vi "Instantiate_llm_azureopenai.vi"(0 "deployement name":string(combo), 5 "azure_endpoint":string, 7 "azure_api_key":string, 9 "api_version":string, 11 "error in (no error)":errorcluster) -> (4 "llm_azureopenai_chatmodels out":refnum<class "llm_azureopenai_chatmodels.lvclass">, 15 "error out":errorcluster)   [LabVIEW 2020, in "llm_azureopenai_chatmodels.lvclass"]
uses:
  llm_azureopenai_chatmodels.lvclass
  D:/Personal/LabVIEW LLMs/src/models/llm_openai_chatmodels/llm_openai_chatmodels.lvclass
  D:/Personal/LabVIEW LLMs/src/models/abstract_llm_base/abstract_llm_base.lvclass
  llm_azureopenai_chatmodels.lvclass/llm_azureopenai_chatmodels.ctl
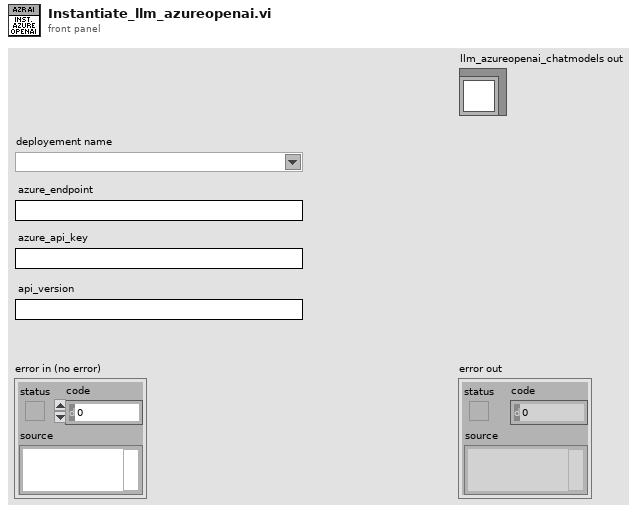
[diagram p1: front panel]
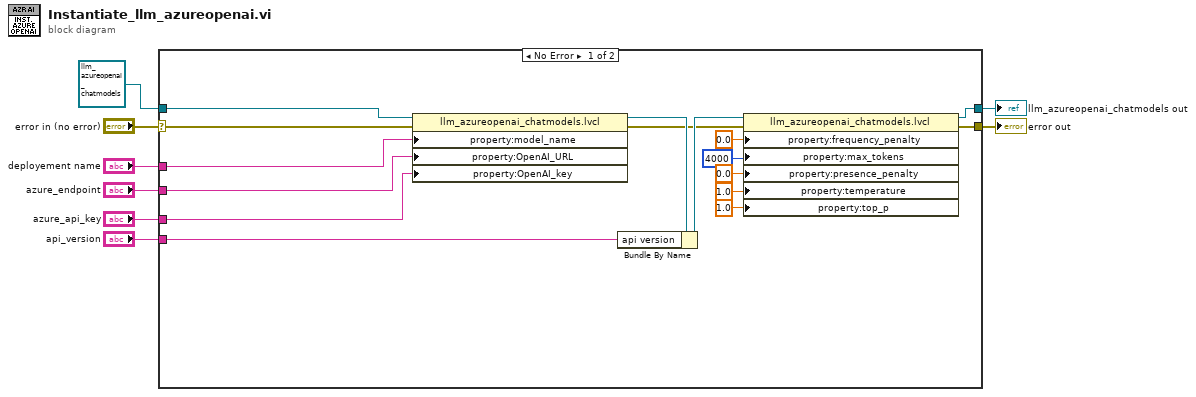
[diagram p0: block diagram]
diagram:
  n1 = case shown="No Error" "error in (no error)" {
    selector: "error in (no error)" -> [w23 w26]
    tunnel: [w10 w26] -> w7
    tunnel: [w9 w25] -> w5
    tunnel: refnum<class "llm_azureopenai_chatmodels.lvclass"> refnum ("llm_azureopenai_chatmodels in") -> [w24 w25]
    tunnel: "deployement name" -> [w22 _]
    tunnel: "azure_endpoint" -> [w21 _]
    tunnel: "azure_api_key" -> [w20 _]
    tunnel: "api_version" -> [w18 _]
    frame No Error {
      n2 = property class="llm_azureopenai_chatmodels.lvcl"(reference=w24, error in=w23, "property:model_name"=w22, "property:OpenAI_URL"=w21, "property:OpenAI_key"=w20) -> (reference out=w19:refnum<class "llm_azureopenai_chatmodels.lvclass">, error out=w11:errorcluster)
      n3 = Bundle By Name(cluster=w19, "api version"=w18) -> (w12:refnum<class "llm_azureopenai_chatmodels.lvclass">)
      n4 = property class="llm_azureopenai_chatmodels.lvcl"(reference=w12, error in=w11, "property:frequency_penalty"=0.0 ("frequency_penalty"), "property:max_tokens"=u32 4000 ("max_tokens"), "property:presence_penalty"=0.0 ("presence_penalty"), "property:temperature"=1.0 ("temperature"), "property:top_p"=1.0 ("top_p")) -> (reference out=w9:refnum<class "llm_azureopenai_chatmodels.lvclass">, error out=w10:errorcluster)
    }
    frame Error {
    }
  }
  "error out" <- w7
  "llm_azureopenai_chatmodels out" <- w5
